vi "Execute Scalar-Mixer ECal.vi"(6 "Port 2  (2)":i32=2, 7 "Channel (1)":i32=1, 8 "error in (no error)":errorcluster, 9 "Port 1 (1)":i32=1, 10 "Calibration (0: 1-port)":u16(ring) items=["1-port", "2-port"], 11 "VISA resource name":refnum<visa-resource-name>) -> (0 "error out":errorcluster, 3 "VISA resource name out":refnum<visa-resource-name>)   [LabVIEW 2022 SP3, in "Agilent ENA Series.lvlib"]
doc: "Performs 1-port or 2-port, for selected channel, ECal module measurement and error coefficient calculation (scalar-mixer calibration) when the frequency offset mode is enabled.\n\n<b>Note:</b>\nThis VI is not supported by the E5063A, E5080A or E5080B."
uses:
  <instrlib>/Agilent ENA Series/Agilent ENA Series.lvlib
panel:
  # "Note:\nThis VI is not supported by the E5063A, E5080A, E5080B."
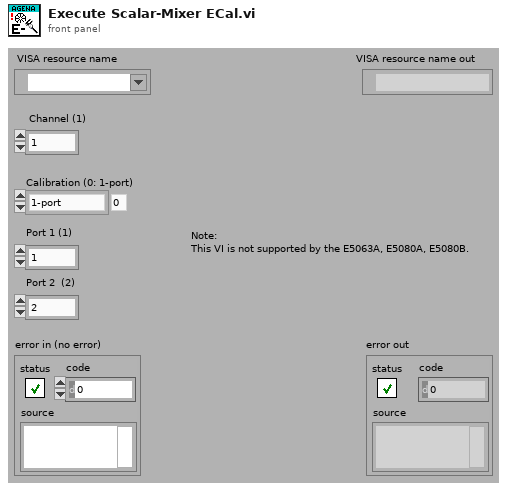
[diagram p1: front panel]
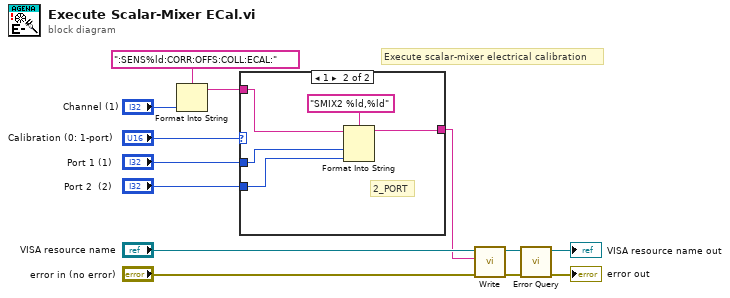
[diagram p0: block diagram]
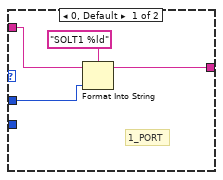
[diagram p2: hidden frame]
diagram:
  # "Execute scalar-mixer electrical calibration"
  n1 = Format Into String(format string=":SENS%ld:CORR:OFFS:COLL:ECAL:", "Channel (1)") -> (resulting string=w7:string)  [unwired: 2 in, 1 out]
  n2 = case shown="1" "Calibration (0: 1-port)" {
    tunnel: "Port 1 (1)" -> [w16 w20]
    tunnel: w7 -> [w15 w21]
    tunnel: [w14 w18] -> w5
    tunnel: "Port 2  (2)" -> [_ w19]
    frame 0, Default {
      # "1_PORT"
      n3 = Format Into String(format string="SOLT1 %ld", initial string=w15, w16) -> (resulting string=w14:string)  [unwired: 1 in, 1 out]
    }
    frame 1 {
      # "2_PORT"
      n4 = Format Into String(format string="SMIX2 %ld,%ld", initial string=w21, w20, w19) -> (resulting string=w18:string)  [unwired: 1 in, 1 out]
    }
  }
  n5 = call <instrlib>:"Write.vi"("error in (no error)"="error in (no error)", "String ()"=w5, "VISA resource name"="VISA resource name") -> ("error out"=w3:errorcluster, "VISA resource name out"=w4:refnum<visa-resource-name>)  [unwired: 6 in, 1 out]
  n6 = call <instrlib>:"Error Query.vi"("error in (no error)"=w3, "VISA resource name"=w4) -> ("error out"=→"error out":errorcluster, "VISA resource name out"=→"VISA resource name out":refnum<visa-resource-name>)  [unwired: 6 in, 2 out]
